vi "TestPolyVI.vi"   [LabVIEW 2019]
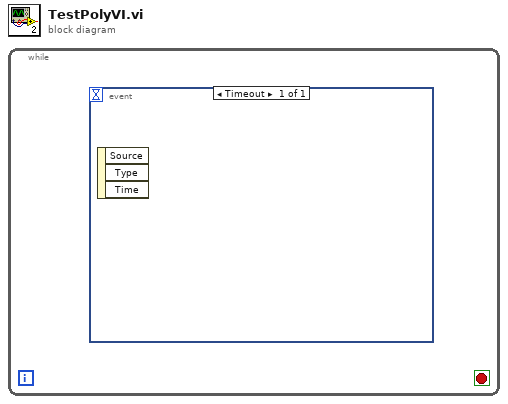
[diagram p0: block diagram]
diagram:
  n1 = while {
    stop <- _ stop-if-true
    n2 = event shown="[0] Timeout" {
      selector: _ -> [_]
      dyn-events: _ -> [_]
      timeout: _ -> [_]
      event Timeout {
        n3 = event-data() -> ()  [unwired: 1 in, 3 out]
      }
    }
  }
